vi "Open Comm.vi"(7 "Serial Configuration":cluster{"Baud Rate":u32}={"Baud Rate"=9600} {"Baud Rate" items=["300"=300, "600"=600, "1200"=1200, "2400"=2400, "4800"=4800, "9600"=9600, "19200"=19200]}, 8 "error in (no error)":errorcluster, 11 "VISA resource in":refnum<visa-resource-name>) -> (0 "error out":errorcluster, 3 "VISA resource out":refnum<visa-resource-name>)   [LabVIEW 2020, in "Global FIA milliGAT.lvlib"]
doc: "Establishes communication with the instrument and optionally performs an instrument identification query and/or an instrument reset. It also places the instrument in a default state needed for other instrument driver operations. Therefore, call this VI before calling other instrument driver VIs for this instrument. Generally, you need to call the <b>Initialize</b> VI only once at the beginning of an application."
uses:
  <instrlib>/RxnRover/Global FIA milliGAT 3.14/Global FIA milliGAT.lvlib
panel:
  # "(c) 2020 Global FIA.  ALL RIGHTS RESERVED."
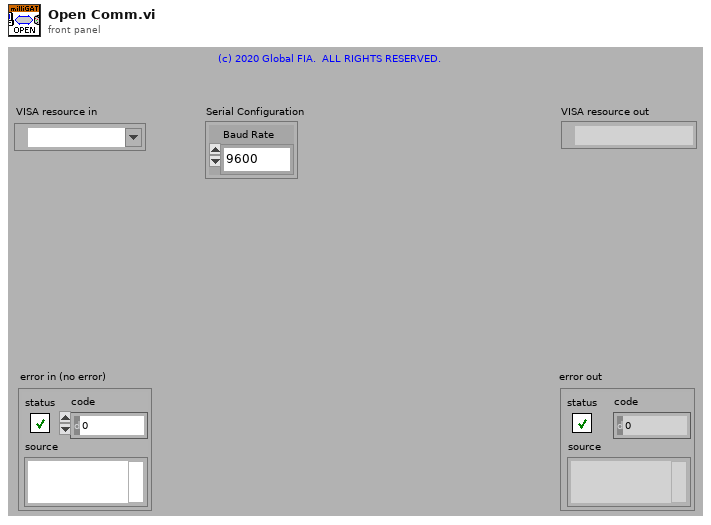
[diagram p1: front panel]
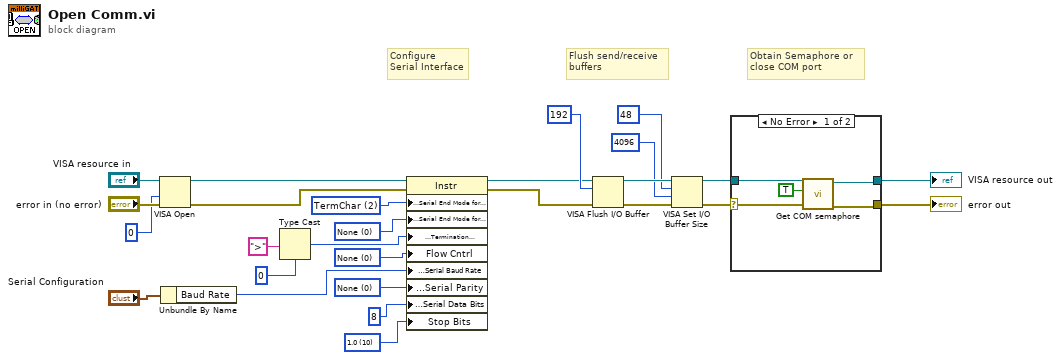
[diagram p0: block diagram]
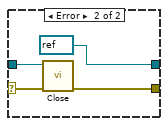
[diagram p2: hidden frame]
diagram:
  w16 = u16 0 items=["None", "XON/XOFF", "RTS/CTS", "XON/XOFF & RTS/CTS", "DTR/DSR", "XON/XOFF & DTR/DSR"] ("Serial Settings:Flow Control")
  w18 = u16 0 items=["None", "Last Bit", "TermChar", "Break"] ("Serial Settings:End Mode for Writes")
  w19 = u16 2 items=["None", "Last Bit", "TermChar"] ("Serial Settings:End Mode for Reads")
  w12 = u16 10 items=["1.0"=10, "1.5"=15, "2.0"=20] ("Serial Settings:Stop Bits")
  w14 = u16 0 items=["None", "Odd", "Even", "Mark", "Space"] ("Serial Settings:Parity")
  # "Obtain Semaphore or\nclose COM port"
  # "Configure\nSerial Interface"
  # "Flush send/receive\nbuffers"
  n1 = VISA Open(access mode=u32 0, error in (no error)="error in (no error)", VISA resource name="VISA resource in") -> (VISA resource name=w11:refnum<visa-resource-name>, error out=w10:errorcluster)  [unwired: 2 in]
  n2 = Unbundle By Name("Serial Configuration") -> ("Baud Rate"=w15:u32)
  n3 = Type Cast(type=u8 0, x=">") -> (*(type *) &x=w17:u8)
  n4 = property on="Property Node" class="Instr"(reference=w11, error in=w10, "Serial Settings:Serial End Mode for Reads"=w19, "Serial Settings:Serial End Mode for Writes"=w18, "Message Based Settings:Termination Character"=w17, "Flow Cntrl"=w16, "Serial Settings:Serial Baud Rate"=w15, "Serial Settings:Serial Parity"=w14, "Serial Settings:Serial Data Bits"=u16 8 ("Serial Settings:Data Bits"), "Stop Bits"=w12) -> (reference out=w4:refnum<visa-resource-name>, error out=w3:errorcluster)
  n5 = VISA Flush I/O Buffer(VISA resource name=w4, mask (16)=u16 192, error in (no error)=w3) -> (VISA resource name out=w9:refnum<visa-resource-name>, error out=w8:errorcluster)
  n6 = VISA Set I/O Buffer Size(VISA resource name=w9, mask (16)=u16 48, size (4096)=u32 4096 ("size (0)"), error in (no error)=w8) -> (VISA resource name out=w2:refnum<visa-resource-name>, error out=w1:errorcluster)
  n7 = case shown="No Error" w1 {
    selector: w1 -> [w29 w34]
    tunnel: w2 -> [w31 w35]
    tunnel: [w30 refnum<visa-resource-name> refnum ("VISA resource out")] -> w25
    tunnel: [w28 w36] -> w24
    frame No Error {
      n8 = call <instrlib>:"Get COM semaphore.vi"("error in (no error)"=w29, "create if not found (T)"=TRUE, "VISA resource in"=w31) -> ("error out"=w28:errorcluster, "VISA resource out"=w30:refnum<visa-resource-name>)  [unwired: 6 in, 1 out]
    }
    frame Error {
      n9 = call <instrlib>:"Close.vi"("error in (no error)"=w34, "VISA resource in"=w35) -> ("error out"=w36:errorcluster)  [unwired: 9 in]
    }
  }
  "VISA resource out" <- w25
  "error out" <- w24
